vi "AWG_send_command.vi"(1 "CMD list":string[](array[string]), 2 "Port number":u16=4000, 3 "IP Address":string) -> ()   [LabVIEW 2013]
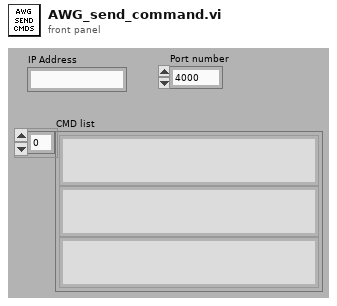
[diagram p1: front panel]
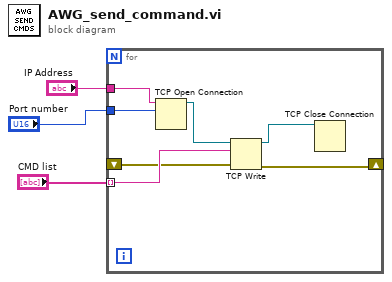
[diagram p0: block diagram]
diagram:
  n1 = for {
    tunnel: "CMD list" -> [w10] mode=indexing
    shift-right: [w5] -> _
    shift-left: _ -> [w6]
    tunnel: "IP Address" -> [w9]
    tunnel: "Port number" -> [w4]
    n2 = TCP Open Connection(address=w9, remote port or service name=w4) -> (connection ID=w8:refnum<k5>)  [unwired: 1 in, 3 out]
    n3 = TCP Write(connection ID=w8, data in=w10, error in (no error)=w6) -> (connection ID out=w7:refnum<k5>, error out=w5:errorcluster)  [unwired: 2 out]
    n4 = TCP Close Connection(connection ID=w7) -> ()  [unwired: 2 in, 2 out]
  }
